vi "写地址转报文.vi"(9 "布尔":bool, 10 "写入触点类型":string, 11 "写入起始地址":string) -> (3 "连接的字符串":string)   [LabVIEW 2018]
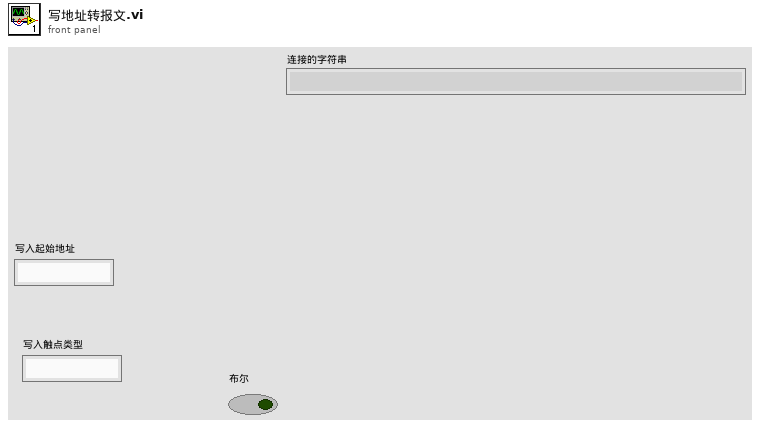
[diagram p1: front panel]
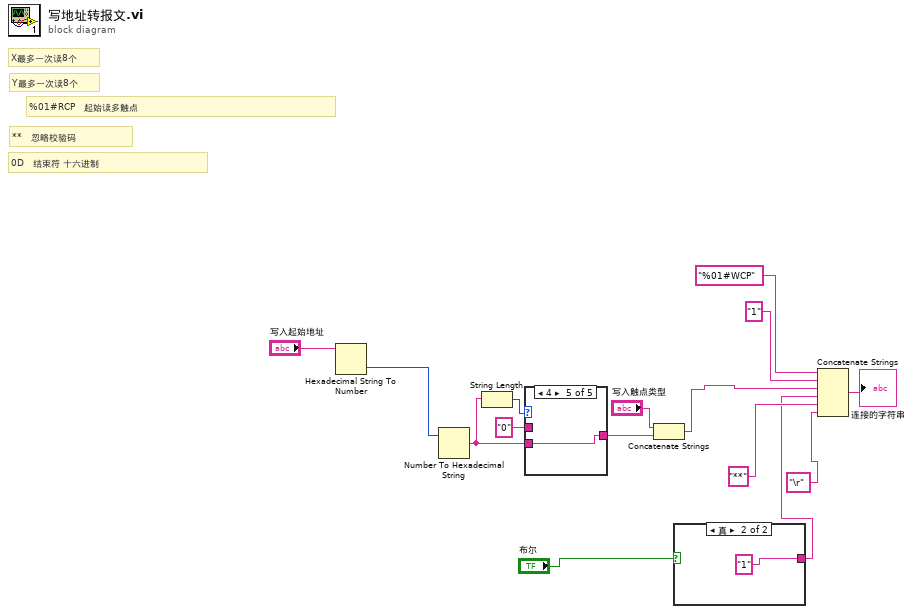
[diagram p0: block diagram]
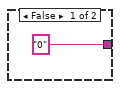
[diagram p2: hidden frame]
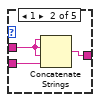
[diagram p4: hidden frame]
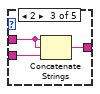
[diagram p5: hidden frame]
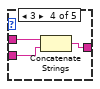
[diagram p6: hidden frame]
diagram:
  # "Y最多一次读8个"
  # "X最多一次读8个"
  # "0D   结束符 十六进制"
  # "**   忽略校验码"
  # "%01#RCP   起始读多触点"
  n1 = Hexadecimal String To Number(string="写入起始地址") -> (number=w11:u32)  [unwired: 2 in, 1 out]
  n2 = Number To Hexadecimal String(2:w11) -> (0:w9:string)  [unwired: 1 in]
  n3 = String Length(string=w9) -> (length=w10:i32)
  n4 = case shown="4" w10 {
    tunnel: w9 -> [w16 w18 w21 w24 w26]
    tunnel: "0" -> [_ w19 w22 w25 _]
    tunnel: [w16 w17 w20 w23 w26] -> w7
    frame 0, Default {
    }
    frame 1 {
      n5 = Concatenate Strings(w19, w19, w19, w18) -> (w17:string)
    }
    frame 2 {
      n6 = Concatenate Strings(w22, w22, w21) -> (w20:string)
    }
    frame 3 {
      n7 = Concatenate Strings(w25, w24) -> (w23:string)
    }
    frame 4 {
    }
  }
  n8 = Concatenate Strings("写入触点类型", w7) -> (w5:string)
  n9 = case shown="真" "布尔" {
    tunnel: ["0" "1"] -> w2
    frame False {
    }
    frame True {
    }
  }
  n10 = Concatenate Strings("%01#WCP" ("字符串"), "1" ("字符串"), w5, w2, "**" ("字符串"), "\r" ("字符串")) -> (→"连接的字符串":string)
